vi "Climb Logic.vi"(8 "Arm Current":dbl, 9 "In Range?":bool, 10 "Limits":cluster{"Base":bool, "Top":bool, "Dummy":bool}, 11 "Climb":bool) -> (0 "Reset Encoder":bool, 1 "Solenoid Value":T1, 2 "Arm Motor":dbl, 3 "Climb State":T2(ring), 4 "Lock":bool, 5 "Arm Set":dbl)   [LabVIEW 2012]
uses:
  <vilib>/Rock Robotics/WPI/Solenoid/WPI_SolenoidValue.ctl
panel:
  out "Numeric":dbl
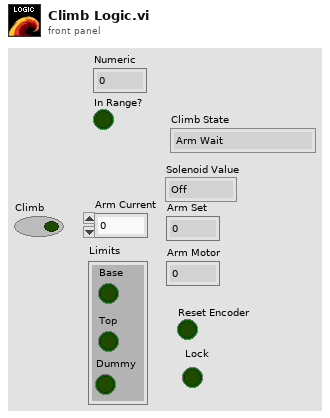
[diagram p1: front panel]
types:
  T1 = typedef "WPI_SolenoidValue.ctl" = enum16{"Off", "On", "Forward", "Reverse"}
  T2 = enum16{"Arm Wait", "Arm Up", "Arm Down", "Arm Attach"}
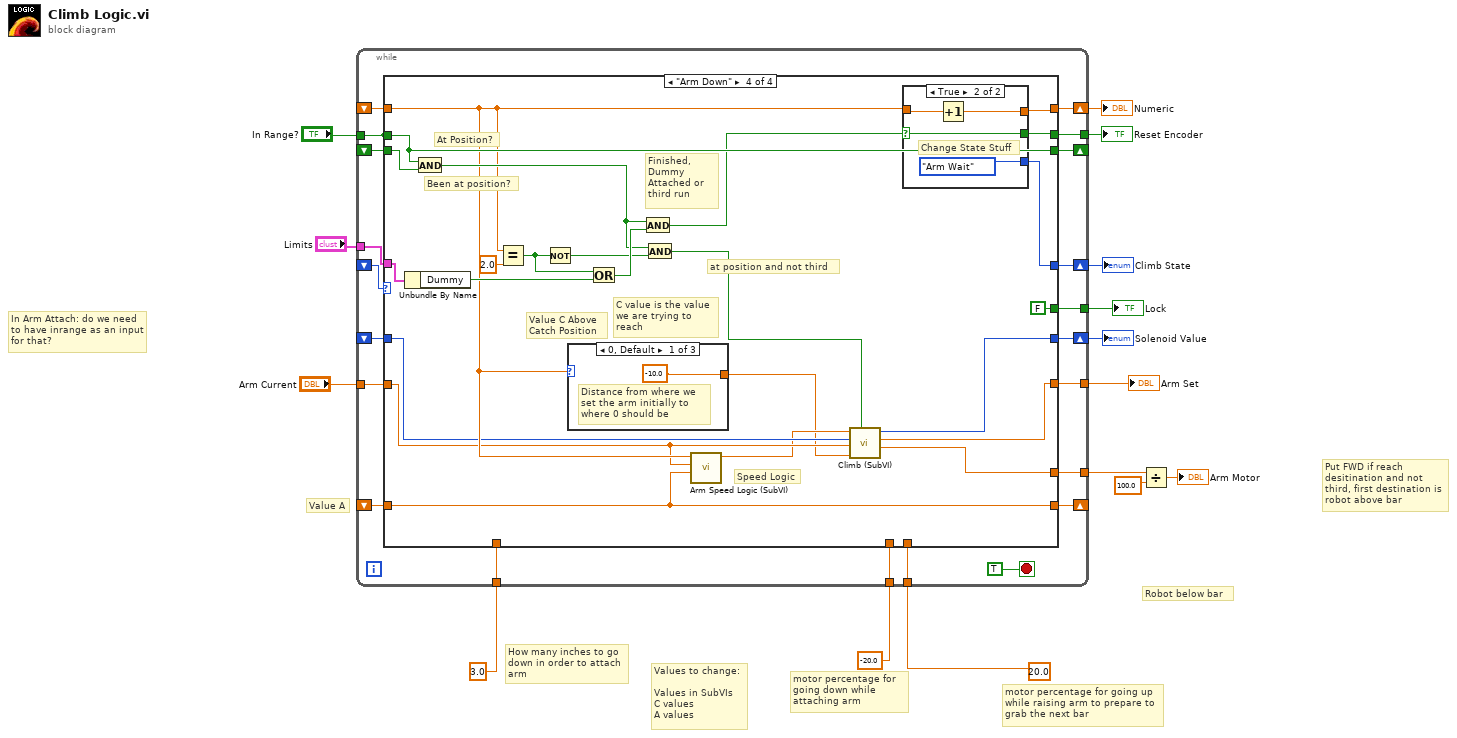
[diagram p0: block diagram]
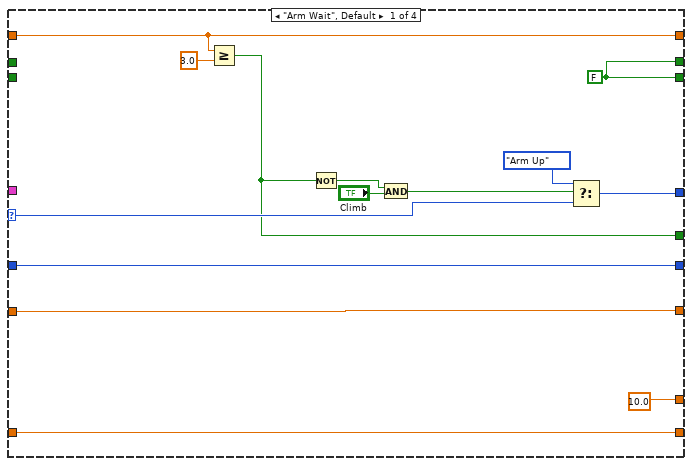
[diagram p2: hidden frame]
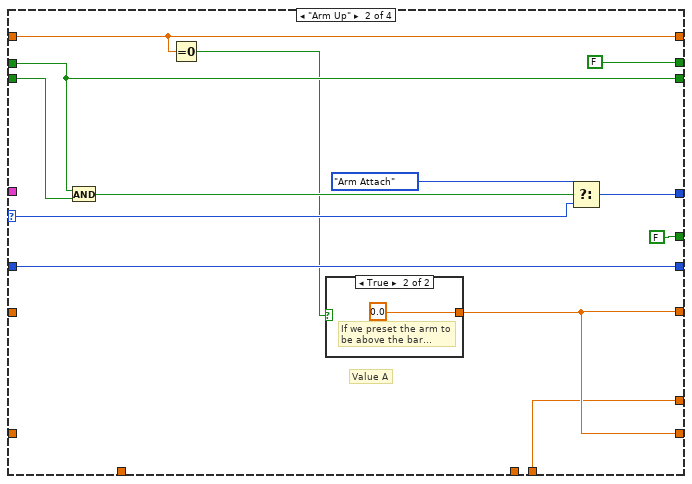
[diagram p3: hidden frame]
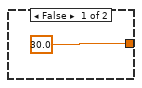
[diagram p4: hidden frame]
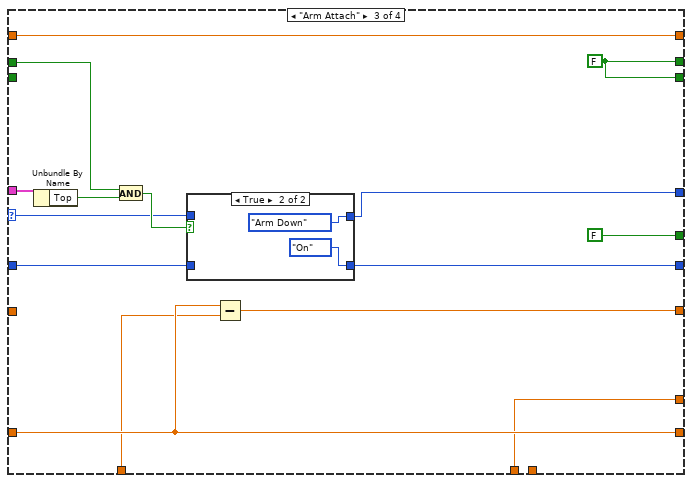
[diagram p5: hidden frame]
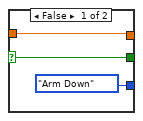
[diagram p7: hidden frame]
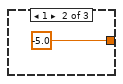
[diagram p8: hidden frame]
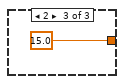
[diagram p9: hidden frame]
diagram:
  # "motor percentage for going up while raising arm to prepare to grab the next bar"
  # "motor percentage for going down while attaching arm"
  # "In Arm Attach: do we need to have inrange as an input for that?"
  # "How many inches to go down in order to attach arm"
  # "Values to change:\n\nValues in SubVIs\nC values\nA values"
  # "Put FWD if reach desitination and not third, first destination is robot above bar"
  # "Robot below bar"
  # "Value A"
  n1 = while {
    shift-right: [w36] -> w11
    shift-left: _ -> [w33]
    tunnel: "In Range?" -> [w20]
    shift-right: [w32] -> _
    shift-left: _ -> [w31]
    tunnel: "Limits" -> [w30]
    shift-right: [w29] -> w12
    shift-left: _ -> [w28]
    tunnel: "Arm Current" -> [w27]
    tunnel: [w34] -> w5
    shift-right: [w26] -> w7
    shift-left: _ -> [w25]
    tunnel: [w24] -> w14
    tunnel: [w23] -> w15
    shift-right: [w22] -> _
    shift-left: _ -> [w21]
    tunnel: [w20] -> _
    tunnel: [w19] -> w8
    tunnel: 3.0 ("y") -> [w18]
    tunnel: -20.0 ("x") -> [w17]
    tunnel: 20.0 ("x") -> [w16]
    stop <- TRUE stop-if-true
    n2 = case shown="\"Arm Down\"" w33 {
      selector: w33 -> [w49 w62 w71 _]
      tunnel: [w50 w63 w69 w91] -> w36
      tunnel: [w47 w52 w77 w89] -> w34
      tunnel: w20 -> [_ w59 w76 w99]
      tunnel: [w46 w59 w74 w99] -> w32
      tunnel: w31 -> [_ w57 _ w98]
      tunnel: w30 -> [_ _ w80 w108]
      tunnel: [w37 w58 w68 w107] -> w29
      tunnel: w28 -> [w37 w58 w70 w88]
      tunnel: w27 -> [w47 _ _ w90]
      tunnel: [w45 w56 w73 w94] -> w26
      tunnel: w25 -> [w45 w56 w73 w93]
      tunnel: [w46 FALSE ("At Position") w74 w92] -> w24
      tunnel: [w38 FALSE FALSE FALSE] -> w23
      tunnel: [w40 w52 w78 w105] -> w22
      tunnel: w21 -> [w40 _ w78 w105]
      tunnel: [10.0 ("x") w51 w66 w104] -> w19
      tunnel: w18 -> [_ _ w67 _]
      tunnel: w17 -> [_ _ w66 _]
      tunnel: w16 -> [_ w51 _ _]
      frame "Arm Wait", Default {
        w46 = FALSE ("At Position")
        n3 = Greater Or Equal?(x=w45, y=3.0) -> (x >= y?=w38:bool)
        n4 = Not(x=w38) -> (.not. x?=w41:bool)
        n5 = And(x=w41, y="Climb") -> (x .and. y?=w42:bool)
        n6 = Select(t=T2."Arm Up", s=w42, f=w49) -> (s? t:f=w50:T2)
      }
      frame "Arm Up" {
        # "Value A"
        n7 = And(x=w59, y=w57) -> (x .and. y?=w60:bool)
        n8 = Equal To 0?(x=w56) -> (x = 0?=w53:bool)
        n9 = case shown="True" w53 {
          tunnel: [30.0 ("y") 0.0 ("y")] -> w52
          frame False {
          }
          frame True {
            # "If we preset the arm to be above the bar..."
          }
        }
        n10 = Select(t=T2."Arm Attach", s=w60, f=w62) -> (s? t:f=w63:T2)
      }
      frame "Arm Attach" {
        w74 = FALSE
        n11 = Unbundle By Name(w80) -> ("Top"=w75:bool)
        n12 = And(x=w76, y=w75) -> (x .and. y?=w72:bool)
        n13 = case shown="True" w72 {
          tunnel: [w82 T2."Arm Down" ("t")] -> w69
          tunnel: w71 -> [w82 _]
          tunnel: [w81 WPI_SolenoidValue."On" ("y")] -> w68
          tunnel: w70 -> [w81 _]
          frame False {
          }
          frame True {
          }
        }
        n14 = Subtract(x=w78, y=w67) -> (x-y=w77:dbl)
      }
      frame "Arm Down" {
        # "C value is the value we are trying to reach"
        # "Speed Logic"
        # "Value C Above Catch Position"
        # "Been at position?"
        # "At Position?"
        # "at position and not third"
        # "Finished, Dummy Attached or third run"
        n15 = Unbundle By Name(w108) -> ("Dummy"=w101:bool)
        n16 = And(x=w99, y=w98) -> (x .and. y?=w97:bool)
        n17 = Equal?(x=w93, y=2.0) -> (x = y?=w100:bool)
        n18 = Not(x=w100) -> (.not. x?=w96:bool)
        n19 = case shown="0, Default" w93 {
          tunnel: [-10.0 ("y") -5.0 ("y") 15.0 ("y")] -> w85
          frame 0, Default {
            # "Distance from where we set the arm initially to where 0 should be"
          }
          frame 1 {
          }
          frame 2 {
          }
        }
        n20 = Or(x=w100, y=w101) -> (x .or. y?=w102:bool)
        n21 = And(x=w97, y=w102) -> (x .and. y?=w95:bool)
        n22 = And(x=w97, y=w96) -> (x .and. y?=w87:bool)
        n23 = call "Arm Speed Logic (SubVI).vi"("y"=w105, "Arm Current"=w90, "Numeric"=w93) -> ("f"=w86:dbl)  [unwired: 8 in]
        n24 = call "Climb (SubVI).vi"("At position and not third"=w87, "C"=w85, "Arm Current"=w90, "Solenoid in"=w88, "Input from Speed logic"=w86) -> ("Arm Motor"=w104:dbl, "Arm Set"=w89:dbl, "Solenoid out"=w107:T1)  [unwired: 4 in]
        n25 = case shown="True" w95 {
          selector: w95 -> [w110 w113]
          tunnel: w93 -> [w111 w114]
          tunnel: [w111 w115] -> w94
          tunnel: [w110 w113] -> w92
          tunnel: [T2."Arm Down" ("t") T2."Arm Wait" ("t")] -> w91
          frame False {
          }
          frame True {
            # "Change State Stuff"
            n26 = Increment(x=w114) -> (x+1=w115:dbl)
          }
        }
      }
    }
  }
  "Arm Set" <- w5
  "Climb State" <- w11
  "Solenoid Value" <- w12
  "Reset Encoder" <- w14
  "Lock" <- w15
  "Numeric" <- w7
  n27 = Divide(x=w8, y=100.0) -> (x/y=→"Arm Motor":dbl)
